vi "StMotor_direction_initial.vi"() -> ()   [LabVIEW 2018]
uses:
  <vilib>/LabVIEW Interface for Arduino/Type Defs/Connection Type.ctl
  <vilib>/LabVIEW Interface for Arduino/LabVIEW Interface for Arduino.lvlib
panel:
  in  "stop":bool
  in  "Stop Reverse movement":bool
  in  "Stop Forward movement":bool
  in  "?":i8(slide) step=1 scale=0.0..2.0
  in  "Stepper #":u8
  in  "VISA resource":refnum<visa-resource-name>
  in  "error in":errorcluster
  out "Steps Remaining?":bool
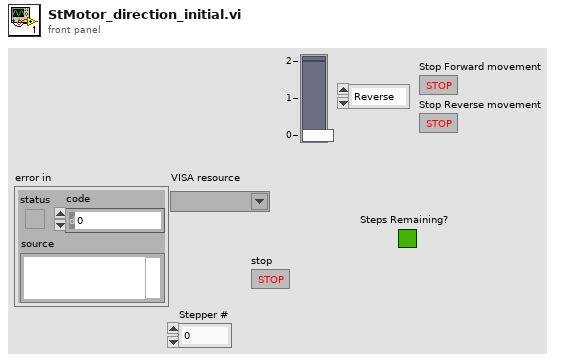
[diagram p1: front panel]
types:
  T1 = typedef "LabVIEW Interface for Arduino.lvlib/Connection Type.ctl" = enum8{"USB / Serial", "XBEE", "BlueSmirf (Bluetooth)"}
  T2 = typedef "LabVIEW Interface for Arduino.lvlib/Arduino Resource.ctl" = cluster{"VISA resource":refnum<visa-resource-name>, "Board Type":T3, "Connection Type":enum8{"USB / Serial"}, "Bytes Per Packet (15)":u8}
  T3 = typedef "LabVIEW Interface for Arduino.lvlib/Board Type.ctl" = enum16{"Uno", "Dimuelanove w/Atmega 328", "Mega 2560"}
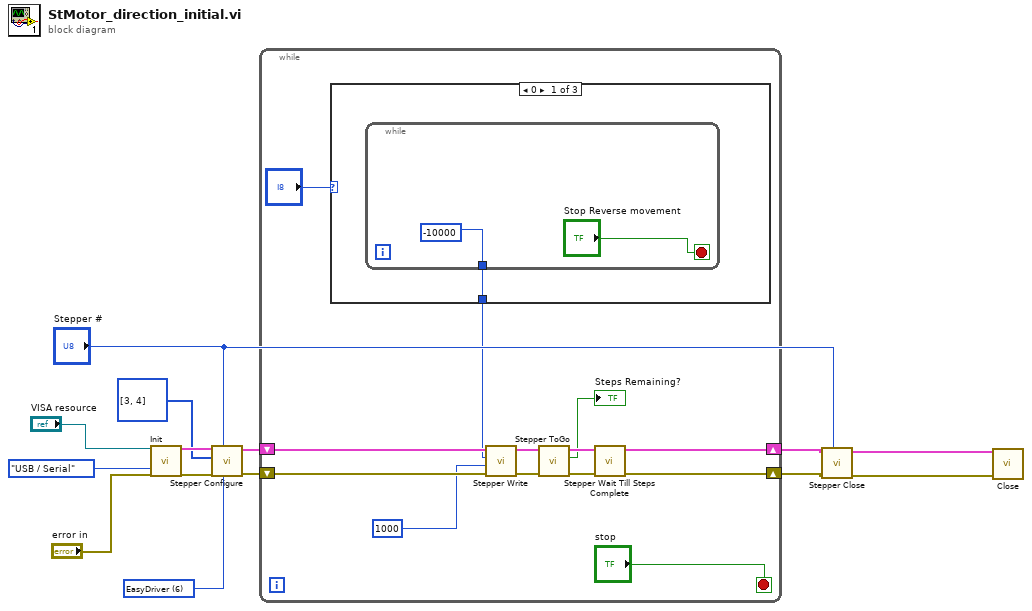
[diagram p0: block diagram]
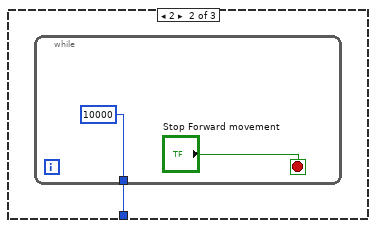
[diagram p2: hidden frame]
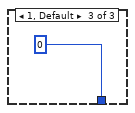
[diagram p3: hidden frame]
diagram:
  w9 = u8 6 items=["2 Wire (Pulse & Direction)"=1, "2 Wire"=2, "4 Wire"=4, "EasyDriver"=6, "AF Motor Shield (Stepper 1 & 2 Only)"=5] ("Control Method")
  n1 = call <vilib>:"Init.vi"("VISA resource"="VISA resource", "Connection Type (USB/Serial)"=Connection_Type."USB / Serial", "error in"="error in") -> ("Arduino Resource"=w13:T2, "error out"=w14:errorcluster)  [unwired: 15 in]
  n2 = call <vilib>:"Stepper Configure.vi"("Control Method"=w9, "Stepper #"="Stepper #", "error in"=w14, "Stepper Pins"=u8[] [3, 4], "Arduino Resource"=w13) -> ("error out"=w6:errorcluster, "Arduino Resource Out"=w7:T2)  [unwired: 5 in]
  n3 = while {
    shift-right: [w17] -> w5
    shift-left: w7 -> [w22]
    shift-right: [w16] -> w4
    shift-left: w6 -> [w21]
    stop <- "stop" stop-if-true
    n4 = case shown="0" "?" {
      tunnel: [w28 w31 i16 0 ("# of Steps to Move")] -> w18
      frame 0 {
        n5 = while {
          tunnel: [i16 -10000 ("# of Steps to Move")] -> w28
          stop <- "Stop Reverse movement" stop-if-true
        }
      }
      frame 2 {
        n6 = while {
          tunnel: [i16 10000 ("# of Steps to Move")] -> w31
          stop <- "Stop Forward movement" stop-if-true
        }
      }
      frame 1, Default {
      }
    }
    n7 = call <vilib>:"Stepper Write.vi"("error in"=w21, "Set Speed (Steps per Second)"=i16 1000, "# of Steps to Move"=w18, "Arduino Resource"=w22) -> ("error out"=w24:errorcluster, "Arduino Resource Out"=w23:T2)  [unwired: 6 in]
    n8 = call <vilib>:"Stepper ToGo.vi"("error in"=w24, "Arduino Resource"=w23) -> ("error out"=w27:errorcluster, "Steps Remaining?"=→"Steps Remaining?":bool, "Arduino Resource Out"=w26:T2)  [unwired: 6 in, 1 out]
    n9 = call <vilib>:"Stepper Wait Till Steps Complete.vi"("error in"=w27, "Arduino Resource In"=w26) -> ("error out"=w16:errorcluster, "Arduino Resource Out"=w17:T2)  [unwired: 8 in]
  }
  n10 = call <vilib>:"Stepper Close.vi"("Stepper #"="Stepper #", "error in"=w4, "Arduino Resource"=w5) -> ("error out"=w2:errorcluster, "Arduino Resource Out"=w3:T2)  [unwired: 7 in]
  n11 = call <vilib>:"Close.vi"("Arduino Resource"=w3, "error in"=w2) -> ()  [unwired: 13 in, 1 out]
